vi "Harv_2_9.vi"(0 "HarvSetpoints":dbl[](array[numeric]), 1 "HarvPot":dbl, 3 "Count":i32, 4 "BallAcquired":bool, 5 "FireBallSen":bool, 6 "Fire":bool, 7 "Harvest":bool, 8 "HPButton":bool, 9 "inAuton?":bool, 10 "WinchDown":bool, 12 "HarvPivUP":bool, 13 "HarvPivPickupLim":bool) -> (14 "HarvPower":dbl, 15 "HarvRoller":dbl, 17 "CountOut":i32, 18 "HarvStart":bool, 19 "HarvCleared":bool)   [LabVIEW 2013]
panel:
  in  "f":dbl
  in  "MotorScale":dbl=1.5
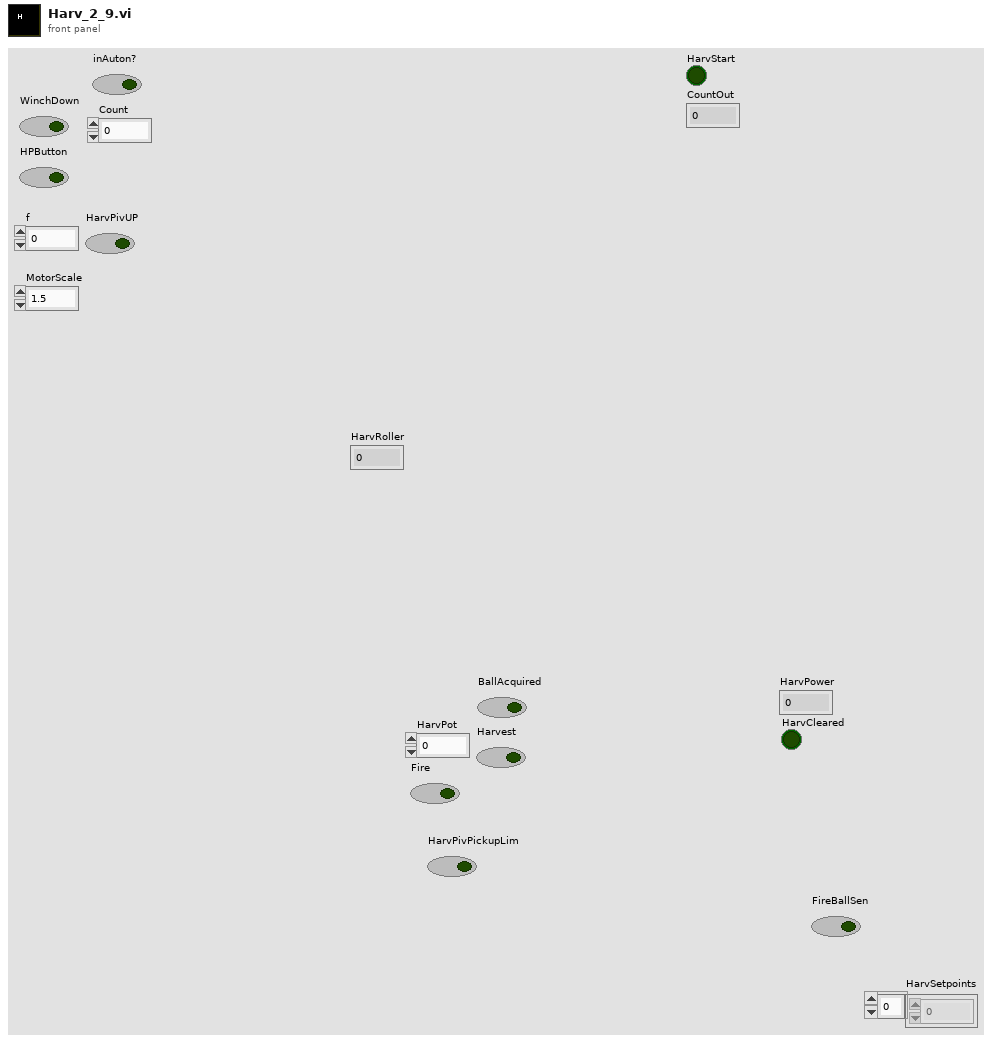
[diagram p1: front panel]
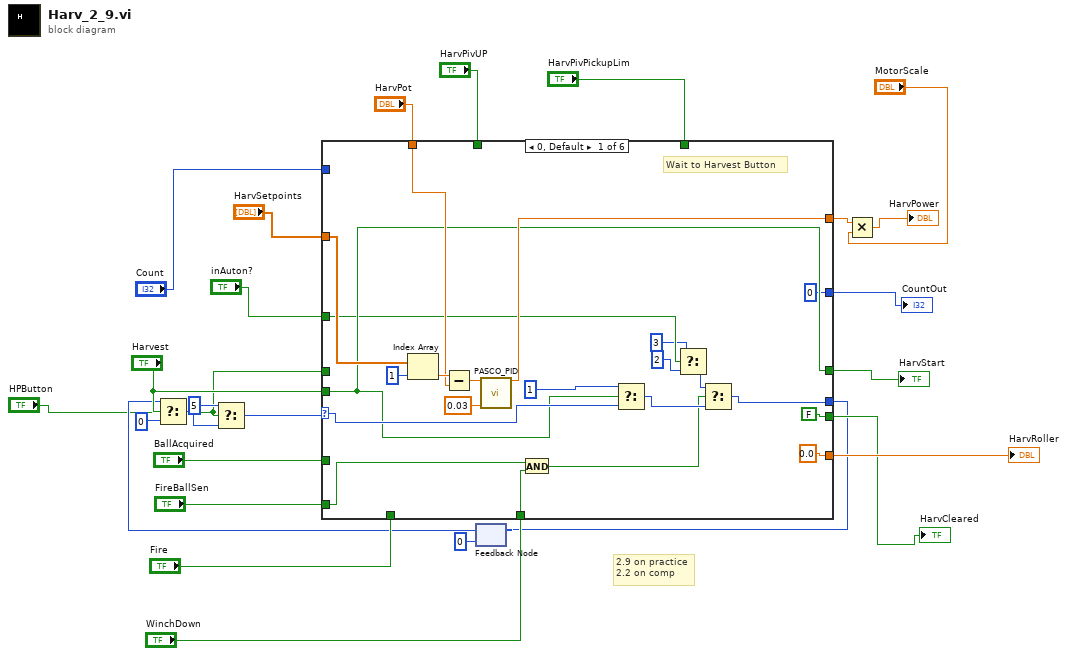
[diagram p0: block diagram]
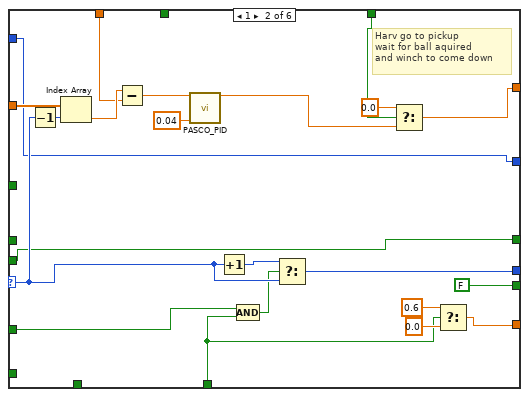
[diagram p2: hidden frame]
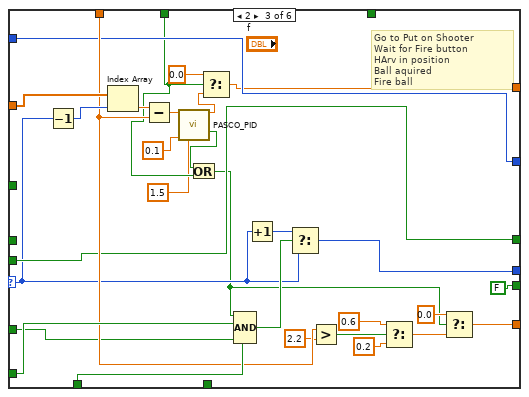
[diagram p3: hidden frame]
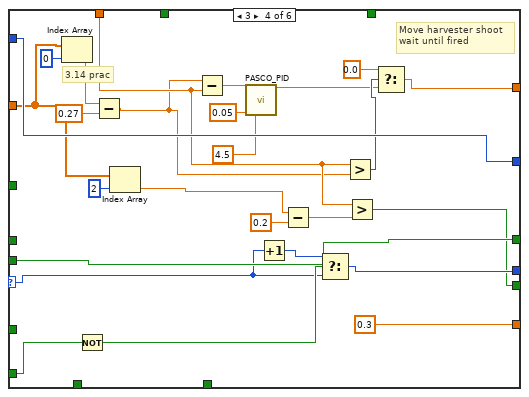
[diagram p4: hidden frame]
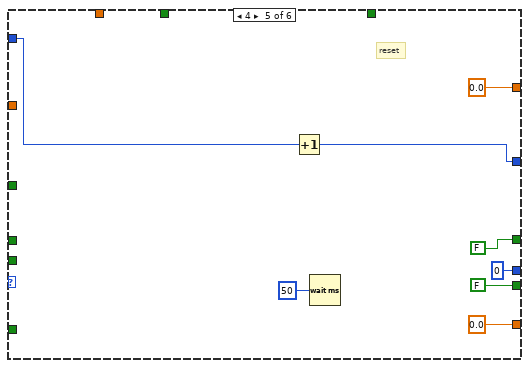
[diagram p5: hidden frame]
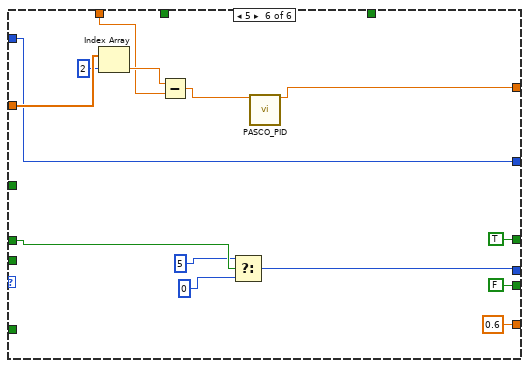
[diagram p6: hidden frame]
diagram:
  # "2.9 on practice\n2.2 on comp"
  n1 = feedback #1(0 ("f")) -> (w19:i32)
  n2 = Select(t=w19, s="Harvest", f=0) -> (s? t:f=w4:i32)
  n3 = Select(t=5, s="HPButton", f=w4) -> (s? t:f=w3:i32)
  n4 = case shown="0, Default" w3 {
    selector: w3 -> [w45 w63 w79 w119 _ _]
    tunnel: "HarvSetpoints" -> [w44 w70 w100 w104 _ w148]
    tunnel: "HarvPot" -> [w43 w68 w91 w109 _ w145]
    tunnel: [w38 w50 w77 w111 0.0 ("Output") w143] -> w18
    tunnel: [w35 w65 w97 w124 0 ("t") w138] -> w8
    tunnel: [0.0 ("f") w57 w84 0.3 ("f") 0.0 ("f") 0.6 ("f")] -> w24
    tunnel: "BallAcquired" -> [_ w59 w81 _ _ _]
    tunnel: "FireBallSen" -> [w33 _ w95 w122 _ _]
    tunnel: "Fire" -> [_ _ w94 _ _ _]
    tunnel: "Harvest" -> [w36 w60 w82 w123 _ _]
    tunnel: [FALSE ("IsThere") FALSE ("IsThere") FALSE ("IsThere") w110 FALSE ("IsThere") FALSE ("IsThere")] -> w15
    tunnel: "HarvPivPickupLim" -> [_ w52 _ _ _ _]
    tunnel: "HarvPivUP" -> [_ _ w73 _ _ _]
    tunnel: [w36 w60 w82 w123 FALSE ("Harvest") TRUE ("Harvest")] -> w12
    tunnel: "WinchDown" -> [w32 w54 _ _ _ _]
    tunnel: "inAuton?" -> [w28 _ _ _ _ _]
    tunnel: [0 ("Count") w53 w78 w118 w128 w142] -> w6
    tunnel: "Count" -> [_ w53 w78 w118 w127 w142]
    tunnel: "HPButton" -> [_ _ _ _ _ w141]
    frame 0, Default {
      # "Wait to Harvest Button"
      n5 = Index Array(array=w44, index=1) -> (element=w46:dbl)
      n6 = Subtract(x=w46, y=w43) -> (x-y=w47:dbl)
      n7 = call "PASCO_PID.vi"("Delta"=w47, "Deadband"=0.03) -> ("Output"=w38:dbl)  [unwired: 12 in, 1 out]
      n8 = And(x=w33, y=w32) -> (x .and. y?=w31:bool)
      n9 = Select(t=1, s=w36, f=w45) -> (s? t:f=w37:i32)
      n10 = Select(t=3, s=w28, f=2 ("t")) -> (s? t:f=w29:i32)
      n11 = Select(t=w29, s=w31, f=w37) -> (s? t:f=w35:i32)
    }
    frame 1 {
      # "Harv go to pickup\nwait for ball aquired\nand winch to come down"
      n12 = Decrement(x=w63) -> (x-1=w64:i32)
      n13 = Index Array(array=w70, index=w64) -> (element=w69:dbl)
      n14 = Subtract(x=w69, y=w68) -> (x-y=w67:dbl)
      n15 = call "PASCO_PID.vi"("Delta"=w67, "Deadband"=0.04) -> ("Output"=w51:dbl)  [unwired: 12 in, 1 out]
      n16 = Increment(x=w63) -> (x+1=w66:i32)
      n17 = Compound Arithmetic op=AND(w59, w54) -> (w58:bool)
      n18 = Select(t=w66, s=w58, f=w63) -> (s? t:f=w65:i32)
      n19 = Select(t=0.0, s=w52, f=w51) -> (s? t:f=w50:dbl)
      n20 = Select(t=0.6, s=w54, f=0.0) -> (s? t:f=w57:dbl)
    }
    frame 2 {
      # "Go to Put on Shooter\nWait for Fire button\nHArv in position\nBall aquired \nFire ball"
      n21 = Decrement(x=w79) -> (x-1=w93:i32)
      n22 = Index Array(array=w100, index=w93) -> (element=w99:dbl)
      n23 = Subtract(x=w99, y=w91) -> (x-y=w98:dbl)
      n24 = call "PASCO_PID.vi"("Delta"=w98, "Deadband"=0.1, "P Gain"=1.5) -> ("Output"=w76:dbl, "IsThere"=w74:bool)  [unwired: 11 in]
      n25 = Or(x=w74, y=w73) -> (x .or. y?=w72:bool)
      n26 = Select(t=0.0, s=w73, f=w76) -> (s? t:f=w77:dbl)
      n27 = Compound Arithmetic op=AND(w72, w95, w94, w81) -> (w96:bool)
      n28 = Increment(x=w79) -> (x+1=w80:i32)
      n29 = Select(t=w80, s=w96, f=w79) -> (s? t:f=w97:i32)
      n30 = Greater?(x=w91, y=2.2) -> (0:w89:bool)
      n31 = Select(t=0.6, s=w89, f=0.2) -> (s? t:f=w85:dbl)
      n32 = Select(t=0.0, s=w72, f=w85) -> (s? t:f=w84:dbl)
    }
    frame 3 {
      # "3.14 prac"
      # "Move harvester shoot\nwait until fired"
      n33 = Index Array(array=w104, index=0) -> (element=w103:dbl)
      n34 = Not(x=w122) -> (.not. x?=w121:bool)
      n35 = Subtract(x=w103, y=0.27) -> (x-y=w102:dbl)
      n36 = Index Array(array=w104, index=2) -> (element=w107:dbl)
      n37 = Subtract(x=w102, y=w109) -> (x-y=w117:dbl)
      n38 = call "PASCO_PID.vi"("Delta"=w117, "Deadband"=0.05, "P Gain"=4.5) -> ("Output"=w112:dbl)  [unwired: 11 in, 1 out]
      n39 = Increment(x=w119) -> (x+1=w120:i32)
      n40 = Subtract(x=w107, y=0.2) -> (x-y=w108:dbl)
      n41 = Select(t=w120, s=w121, f=w119) -> (s? t:f=w124:i32)
      n42 = Greater?(x=w109, y=w102) -> (0:w114:bool)
      n43 = Greater?(x=w109, y=w108) -> (0:w110:bool)
      n44 = Select(t=0.0, s=w114, f=w112) -> (s? t:f=w111:dbl)
    }
    frame 4 {
      # "reset"
      n45 = Increment(x=w127) -> (x+1=w128:i32)
      n46 = Wait (ms)(milliseconds to wait=u32 50) -> ()  [unwired: 1 out]
    }
    frame 5 {
      n47 = Index Array(array=w148, index=2) -> (element=w146:dbl)
      n48 = Subtract(x=w146, y=w145) -> (x-y=w144:dbl)
      n49 = Select(t=5 ("index"), s=w141, f=0 ("index")) -> (s? t:f=w138:i32)
      n50 = call "PASCO_PID.vi"("Delta"=w144) -> ("Output"=w143:dbl)  [unwired: 13 in, 1 out]
    }
  }
  "HarvRoller" <- w24
  "HarvCleared" <- w15
  "HarvStart" <- w12
  "CountOut" <- w6
  n51 = feedback-in #1(w8) -> ()
  n52 = Multiply(x=w18, y="MotorScale") -> (x*y=→"HarvPower":dbl)
